vi "Measurement UI.vi"() -> ()   [LabVIEW 2025, in "CAN-LIN Raw Bus Capture UI.lvlib"]
uses:
  CAN-LIN Raw Bus Capture UI.lvlib
  Toggle.ctl
  <vilib>/gRPC/LabVIEW gRPC Library/Shared/grpcId.ctl
  Get Status.vi
  Flush Table.vi
  Create Buffer.vi
  Destroy Table Buffer.vi
  OOB gRPC Client/OOB gRPC Client.lvlib
  <vilib>/gRPC/LabVIEW gRPC Library/grpc-lvsupport-release.lvlib
panel:
  out "New root item?":bool
  in  "Tree Data":string[][](array[string])
  in  "Mapping done?":bool
  in  "Table map":map{string, i32}(c390)
  in  "XNET Sessions map":map{u32, refnum<k21>}(c390)
  in  "Tags map":map{string, bool}(c390)
  out "Valid DBC file?":bool
  out "Signals in DBC":i32
  out "Frames in DBC":i32
  in  "Frames Map":map{u32, refnum<k21>}(c390)
  in  "Signals Map":map{u32, refnum<k21>[]}(c390)
  in  "Tree and Table":enum32{"Trace window", "Signal table"}(tab)
  out "Frames":string(tree)
  out "Signals":string[][](table)
  in  "HELP":bool
  out "IsRestarting?":bool
  out "Table Buffer":i32
  out "Error (Logic)":string
  out "Status Message":string
  in  "SAVE FORMAT":u16(ring) items=["TDMS", "CSV"]
  out "Connection":bool
  in  "Clear Trace":bool
  in  "Bus Type":string="CAN"
  in  "Lin Interface":string
  in  "Can Interface":string
  in  "PauseResume":bool
  in  "Path":path
  in  "Save":bool
  in  "Filter":string
  in  "SortByID":bool
  out "Status":string
  in  "SETTINGS":enum32{"CAN", "LIN"}(tab)
  in  "IO Mode":enum32{"CAN", "CAN FD", "CAN FD + BRS"}(ring)
  in  "FD ISO Mode":enum32{"ISO", "Non ISO", "Legacy ISO"}(ring)
  in  "Baudrate":u32=125000
  in  "FD Baudrate":u32=1000000
  in  "Termination CAN":T1
  in  "INTERFACE NAME CAN":refnum<k21>
  in  "DBC path":path
  in  "Termination LIN":T1
  in  "INTERFACE NAME LIN":refnum<k21>
  out "Buffer Size":i32
  out "OOB gRPC Port":i32
  # "CONFIGURATION"
  # "CONTROL"
  # "DBC INFORMATION"
  # "STATUS"
  # "CAN Settings"
  # "LIN Settings"
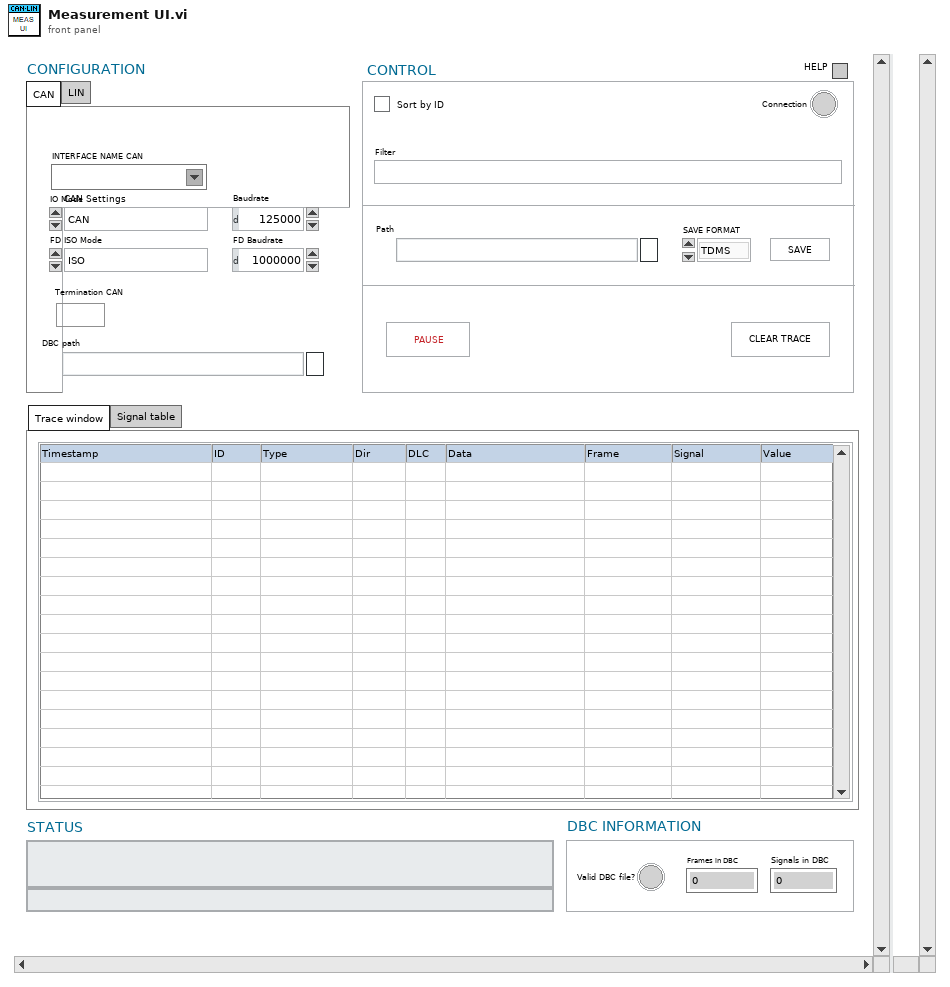
[diagram p1: front panel]
types:
  T1 = typedef "Toggle.ctl" = bool
  T2 = typedef "grpc-lvsupport-release.lvlib/grpcId.ctl" = u64
  T3 = cluster{"New root item?":refnum<vi>, "Tree Data":refnum<vi>, "Mapping done?":refnum<vi>, "Table map":refnum<vi>, "Tags map":refnum<vi>, "XNET Sessions map":refnum<vi>, "Signals":refnum<vi>, "PauseResume":refnum<vi>, "Clear Trace":refnum<vi>, "Path":refnum<vi>, "SAVE FORMAT":refnum<vi>, "Save":refnum<vi>, "Bus Type":refnum<vi>, "Filter":refnum<vi>, "SortByID":refnum<vi>, "Status Message":refnum<vi>, "Frames":refnum<vi>, "DBC path":refnum<vi>, "Signals Map":refnum<vi>, "Frames Map":refnum<vi>, "Frames in DBC":refnum<vi>, "Signals in DBC":refnum<vi>, "Valid DBC file?":refnum<vi>}
  T4 = enum32{"Page Enabled", "Page Disabled", "Page Disabled & Grayed"}
  T5 = enum8{"Enabled", "Disabled", "Disabled and Grayed Out"}
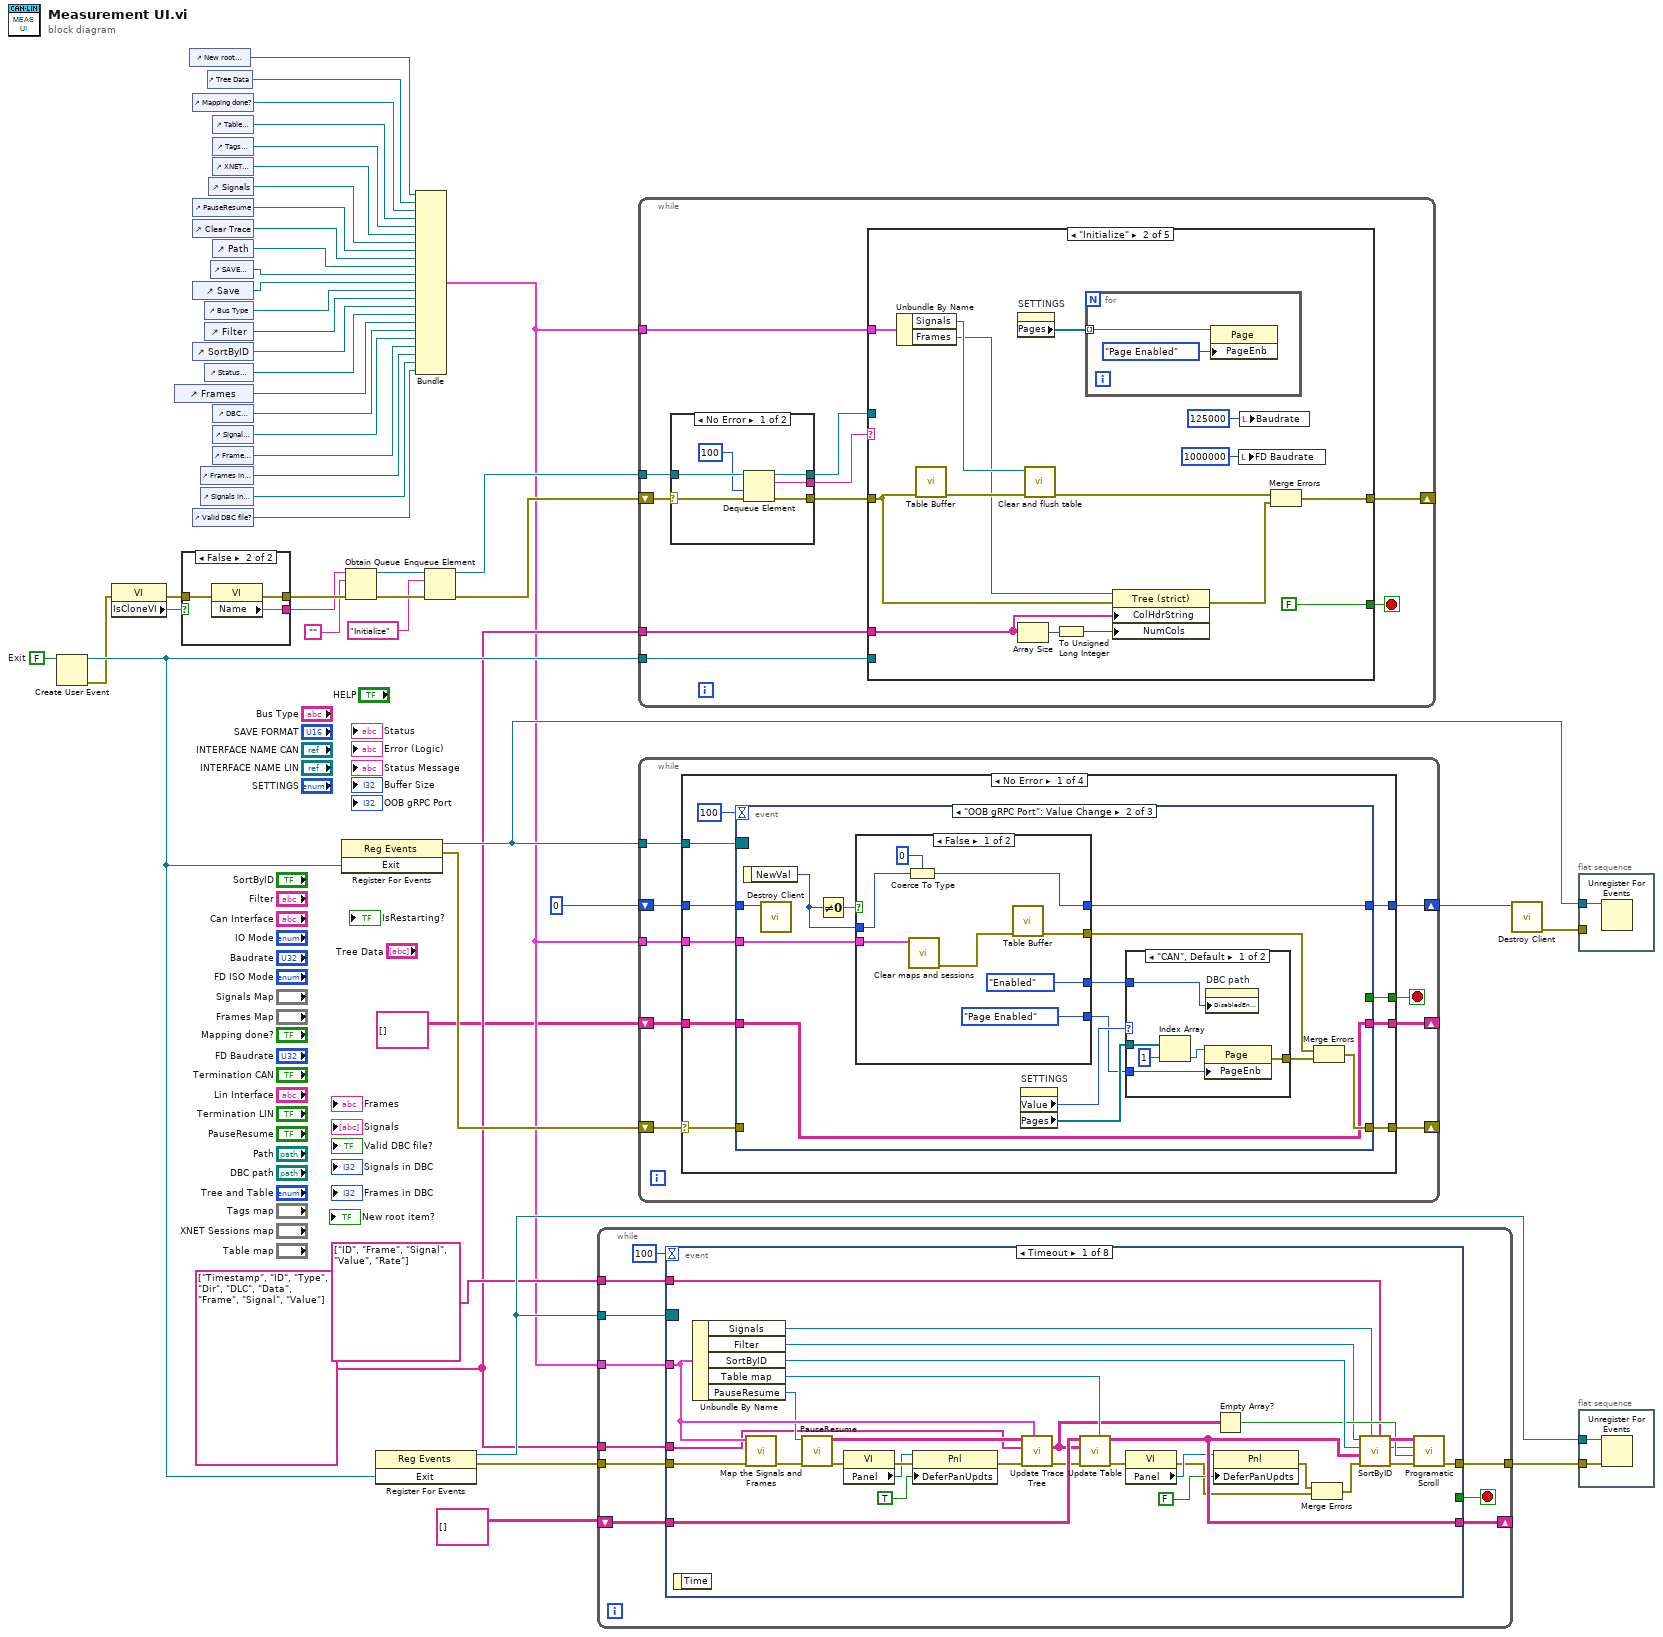
[diagram p0: block diagram]
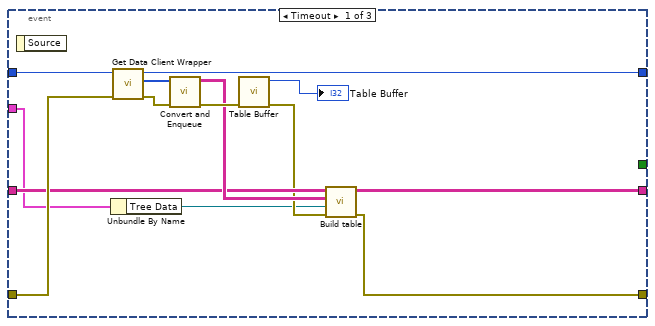
[diagram p2: hidden frame]
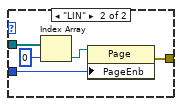
[diagram p3: hidden frame]
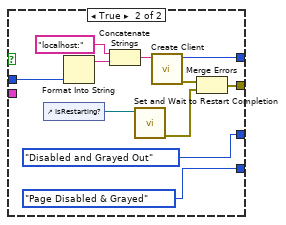
[diagram p4: hidden frame]
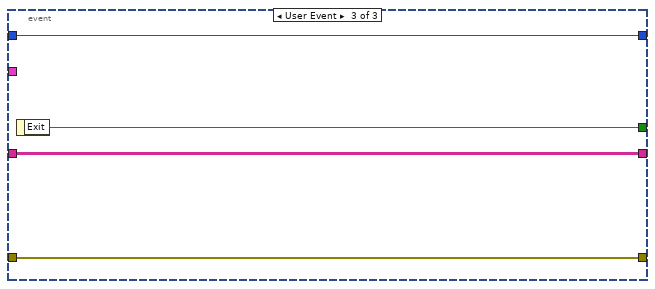
[diagram p5: hidden frame]
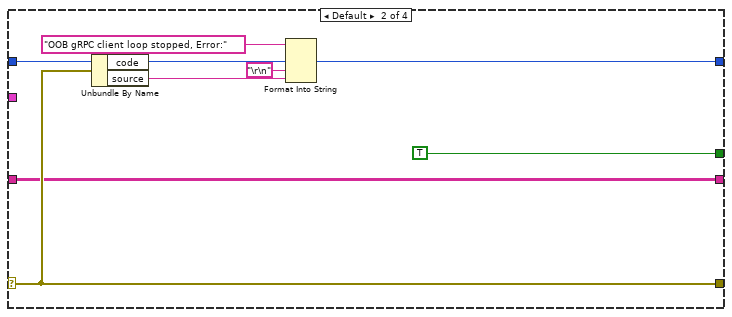
[diagram p6: hidden frame]
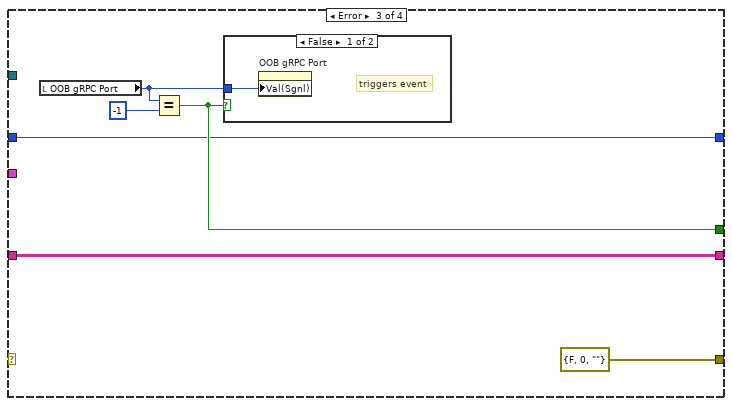
[diagram p7: hidden frame]
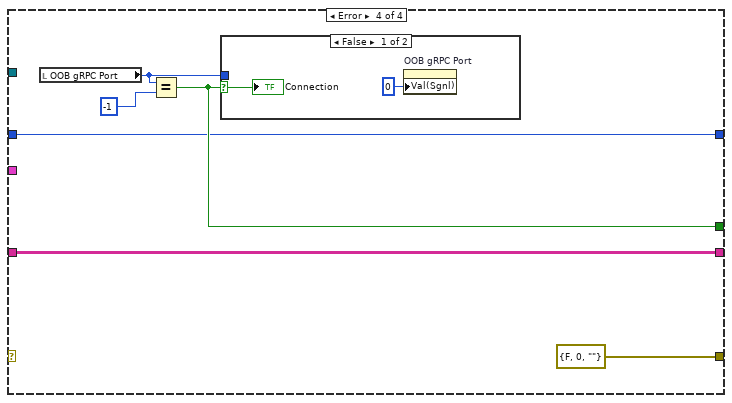
[diagram p9: hidden frame]
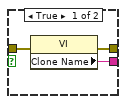
[diagram p11: hidden frame]
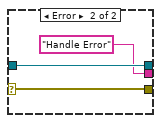
[diagram p12: hidden frame]
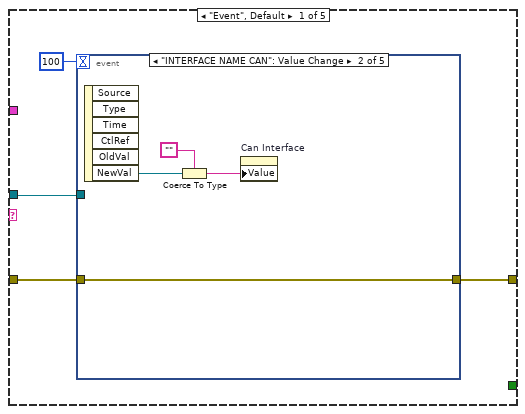
[diagram p13: hidden frame]
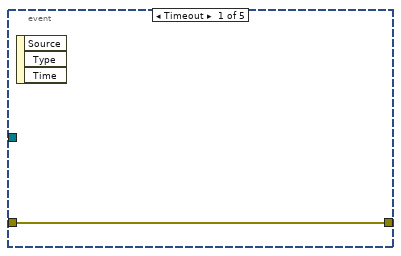
[diagram p14: hidden frame]
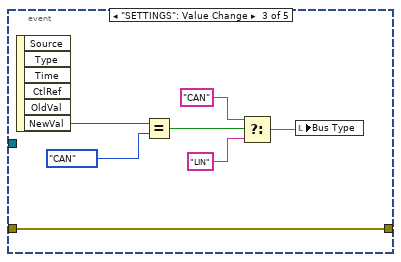
[diagram p15: hidden frame]
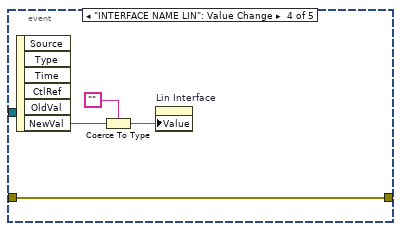
[diagram p16: hidden frame]
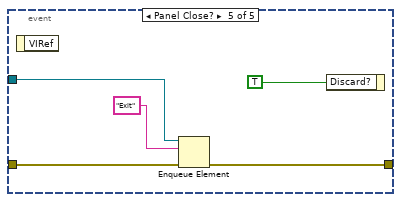
[diagram p17: hidden frame]
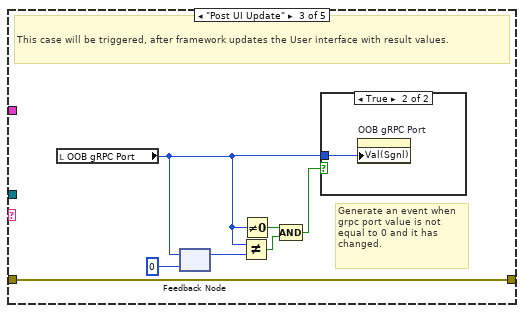
[diagram p18: hidden frame]
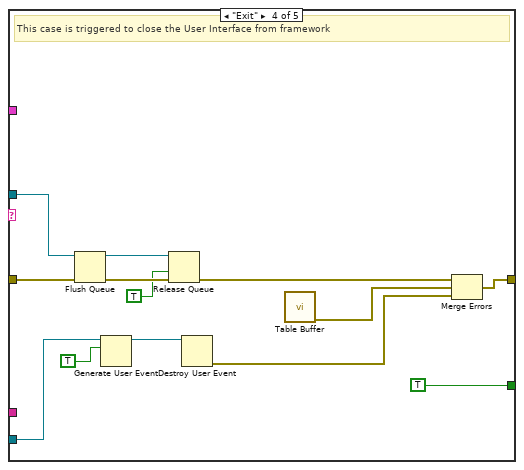
[diagram p20: hidden frame]
diagram:
  w17 = string[] ["Timestamp", "ID", "Type", "Dir", "DLC", "Data", "Frame", "Signal", "Value"] ("Headers")
  w41 = FALSE  # Exit
  n1 = Create User Event(user event datatype=w41) -> (user event=w35:refnum<user-event>, error out=w7:errorcluster)  [unwired: 1 in]
  n2 = property class="VI"(error in=w7) -> (error out=w42:errorcluster, "IsCloneVI"=w43:bool)  [unwired: 1 in, 1 out]
  n3 = control-ref of="Frames"() -> (w21:refnum<vi>)
  n4 = case shown="False" w43 {
    tunnel: [w52 w55] -> w49
    tunnel: [w51 w54] -> w48
    tunnel: w42 -> [w50 w53]
    frame True {
      n5 = property class="VI"(error in=w50) -> (error out=w52:errorcluster, "Clone Name"=w51:string)  [unwired: 1 in, 1 out]
    }
    frame False {
      n6 = property class="VI"(error in=w53) -> (error out=w55:errorcluster, "Name"=w54:string)  [unwired: 1 in, 1 out]
    }
  }
  n7 = control-ref of="New root item?"() -> (w1:refnum<vi>)
  n8 = control-ref of="Mapping done?"() -> (w5:refnum<vi>)
  n9 = control-ref of="PauseResume"() -> (w25:refnum<vi>)
  n10 = control-ref of="Clear Trace"() -> (w33:refnum<vi>)
  n11 = control-ref of="Save"() -> (w30:refnum<vi>)
  n12 = control-ref of="SortByID"() -> (w28:refnum<vi>)
  n13 = control-ref of="Valid DBC file?"() -> (w13:refnum<vi>)
  n14 = control-ref of="Frames in DBC"() -> (w15:refnum<vi>)
  n15 = control-ref of="Signals in DBC"() -> (w14:refnum<vi>)
  n16 = control-ref of="Bus Type"() -> (w29:refnum<vi>)
  n17 = control-ref of="Filter"() -> (w27:refnum<vi>)
  n18 = control-ref of="Status Message"() -> (w26:refnum<vi>)
  n19 = control-ref of="Tree Data"() -> (w2:refnum<vi>)
  n20 = control-ref of="Signals"() -> (w34:refnum<vi>)
  n21 = control-ref of="SAVE FORMAT"() -> (w31:refnum<vi>)
  n22 = control-ref of="Table map"() -> (w10:refnum<vi>)
  n23 = control-ref of="Tags map"() -> (w12:refnum<vi>)
  n24 = control-ref of="XNET Sessions map"() -> (w11:refnum<vi>)
  n25 = control-ref of="Path"() -> (w32:refnum<vi>)
  n26 = control-ref of="DBC path"() -> (w22:refnum<vi>)
  n27 = control-ref of="Signals Map"() -> (w18:refnum<vi>)
  n28 = control-ref of="Frames Map"() -> (w19:refnum<vi>)
  n29 = register-events(w35) -> (reference out=w37:refnum<event-registration>, error out=w40:errorcluster)  [unwired: 2 in]
  n30 = Obtain Queue(name (unnamed)=w48, element data type="", error in (no error)=w49) -> (queue out=w46:refnum<queue>, error out=w47:errorcluster)  [unwired: 2 in, 1 out]
  n31 = register-events(w35) -> (reference out=w24:refnum<event-registration>, error out=w8:errorcluster)  [unwired: 2 in]
  n32 = Bundle("New root item?"=w1, "Tree Data"=w2, "Mapping done?"=w5, "Table map"=w10, "Tags map"=w12, "XNET Sessions map"=w11, "Signals"=w34, "PauseResume"=w25, "Clear Trace"=w33, "Path"=w32, "SAVE FORMAT"=w31, "Save"=w30, "Bus Type"=w29, "Filter"=w27, "SortByID"=w28, "Status Message"=w26, "Frames"=w21, "DBC path"=w22, "Signals Map"=w18, "Frames Map"=w19, "Frames in DBC"=w15, "Signals in DBC"=w14, "Valid DBC file?"=w13) -> (w4:T3)  [unwired: 1 in]
  n33 = Enqueue Element(queue=w46, element="Initialize", error in (no error)=w47) -> (queue out=w16:refnum<queue>, error out=w9:errorcluster)  [unwired: 1 in, 1 out]
  n34 = while {
    tunnel: w8 -> [w65]
    tunnel: [w60] -> w6
    tunnel: w24 -> [w64]
    tunnel: w4 -> [w61]
    shift-right: [w58] -> _
    shift-left: string[][] [] ("Table Data out") -> [w59]
    tunnel: string[] ["ID", "Frame", "Signal", "Value", "Rate"] ("Signal Table Headers") -> [w57]
    tunnel: w17 -> [w56]
    stop <- w63 stop-if-true
    n35 = event shown="[0] Timeout" {
      selector: w64 -> [_ _ _ _ _ _ _ _]
      dyn-events: _ -> [_ _ _ _ _ _ _ _]
      timeout: 100 -> [_ _ _ _ _ _ _ _]
      tunnel: w65 -> [w87 w98 w117 w134 w158 w163 w173 w175]
      tunnel: [w71 w97 w116 w133 w151 w161 w172 w175] -> w60
      tunnel: [_ _ _ _ _ _ _ w176] -> w63
      tunnel: w61 -> [w85 _ w113 w135 w160 w167 _ _]
      tunnel: w59 -> [w82 w96 w108 w132 w155 w168 w171 w174]
      tunnel: [w95 w96 w109 w132 w155 w168 w171 w174] -> w58
      tunnel: w57 -> [w88 _ _ _ w154 _ _ _]
      tunnel: w56 -> [w69 _ _ w130 _ w162 _ _]
      event Timeout {
        n36 = event-data() -> ()  [unwired: 1 in, 1 out]
        n37 = Unbundle By Name(w85) -> ("Signals"=w90:refnum<vi>, "Filter"=w72:refnum<vi>, "SortByID"=w92:refnum<vi>, "Table map"=w83:refnum<vi>, "PauseResume"=w84:refnum<vi>)
        n38 = call "Map the Signals and Frames.vi"("error in"=w87, "References"=w85) -> ("error out"=w86:errorcluster)  [unwired: 9 in]
        n39 = call "PauseResume.vi"("error in"=w86, "PauseResume Ref"=w84) -> ("error out"=w80:errorcluster, "Data"=w89:string[][])  [unwired: 8 in]
        n40 = property class="VI"(error in=w80) -> (error out=w81:errorcluster, "Panel"=w77:refnum<vi>)  [unwired: 1 in, 1 out]
        n41 = property class="Pnl"(reference=w77, error in=w81, "DeferPanUpdts"=TRUE ("Defer Panel Updates")) -> (error out=w79:errorcluster)  [unwired: 1 out]
        n42 = call "Update Trace Tree.vi"("References"=w85, "error in"=w79, "Headers"=w69, "Data IN"=w89) -> ("error out"=w73:errorcluster, "Signals"=w76:string[][])  [unwired: 6 in]
        n43 = call "Update Table.vi"("Table map"=w83, "error in"=w73, "New Data in"=w76, "Table Data in"=w82) -> ("error out"=w70:errorcluster, "Table Data out"=w95:string[][])  [unwired: 6 in]
        n44 = property class="VI"(error in=w70) -> (error out=w68:errorcluster, "Panel"=w74:refnum<vi>)  [unwired: 1 in, 1 out]
        n45 = property class="Pnl"(reference=w74, "DeferPanUpdts"=FALSE ("Defer Panel Updates")) -> (error out=w67:errorcluster)  [unwired: 1 in, 1 out]
        n46 = Empty Array?(array=w76) -> (empty?=w91:bool)
        n47 = Merge Errors(w67, w68) -> (w66:errorcluster)
        n48 = call "SortByID.vi"("Headers"=w88, "Signals table"=w90, "error in"=w66, "Unsorted Data"=w95, "SortByID"=w92, "Filter"=w72) -> ("error out"=w94:errorcluster, "Table Control"=w93:string[][])  [unwired: 4 in]
        n49 = call "Programatic Scroll.vi"("error in"=w94, "Pause? (F)"=w91, "Table Ref"=w90, "Trace"=w93) -> ("error out"=w71:errorcluster)  [unwired: 7 in]
      }
      event "Clear Trace": Value Change {
        # "Run when restarting or then button is pressed down."
        n50 = event-data() -> ("NewVal"=w99:bool)  [unwired: 1 in]
        n51 = case shown="False" w99 {
          tunnel: w98 -> [w102 w103]
          tunnel: [w100 w103] -> w97
          frame False {
            n52 = property on="IsRestarting?" class="Bool (strict)"(error in=w102, "Val(Sgnl)"=FALSE ("Value (Signaling)")) -> (error out=w100:errorcluster)  [unwired: 1 in, 1 out]
          }
          frame True {
          }
        }
      }
      event "IsRestarting?": Value Change {
        n53 = event-data() -> ("NewVal"=w115:bool)  [unwired: 1 in]
        n54 = Unbundle By Name(w113) -> ("Table map"=w104:refnum<vi>, "Tags map"=w105:refnum<vi>, "Frames"=w106:refnum<vi>, "Status Message"=w110:refnum<vi>, "Signals"=w112:refnum<vi>)
        n55 = Not(x=w115) -> (.not. x?=w114:bool)
        n56 = call "Clear Table.vi"("error in"=w117, "Confirm? (F)"=w114, "Table in"=w112) -> ("error out"=w111:errorcluster, "T button?"=w107:bool)  [unwired: 7 in]
        n57 = case shown="True" w107 {
          tunnel: [w119 w128] -> w116
          tunnel: w111 -> [w119 w126]
          tunnel: w110 -> [_ w125]
          tunnel: [w118 string[][] [] ("Table Data out")] -> w109
          tunnel: w108 -> [w118 _]
          tunnel: w106 -> [_ w122]
          tunnel: w105 -> [_ w121]
          tunnel: w104 -> [_ w120]
          frame False {
          }
          frame True {
            # "Reset Table when necessary"
            n58 = invoke class="Map (strict)" method="Reinit To Default"(reference=w120) -> ()  [unwired: 2 in, 3 out]
            n59 = invoke class="Map (strict)" method="Reinit To Default"(reference=w121) -> ()  [unwired: 2 in, 3 out]
            n60 = property class="Str"(reference=w125, error in=w126, "Value"="") -> (error out=w127:errorcluster)  [unwired: 1 out]
            n61 = property on="IsRestarting?" class="Bool (strict)"(error in=w127, "Value"=FALSE ("IsRestarting?")) -> (error out=w128:errorcluster)  [unwired: 1 in, 1 out]
            n62 = invoke on="Invoke Node" class="Tree (strict)" method="Edit Tree Items.Delete"(reference=w122) -> ()  [unwired: 4 in, 5 out]
          }
        }
      }
      event "Save": Value Change {
        n63 = event-data() -> ("NewVal"=w131:bool)  [unwired: 1 in]
        n64 = case shown="False" w131 {
          tunnel: w135 -> [_ w149]
          tunnel: w134 -> [w136 w145]
          tunnel: [w136 w143] -> w133
          tunnel: w130 -> [_ w141]
          frame True {
          }
          frame False {
            n65 = Unbundle By Name(w149) -> ("DBC path"=w138:refnum<vi>, "Status Message"=w140:refnum<vi>, "Path"=w148:refnum<vi>, "SAVE FORMAT"=w147:refnum<vi>, "Bus Type"=w146:refnum<vi>, "Tree Data"=w137:refnum<vi>, "Frames"=w139:refnum<vi>)
            n66 = call "Save CAN data.vi"("Frames"=w139, "DBC path"=w138, "Tree Data"=w137, "Headers"=w141, "error in"=w145, "Bus Type"=w146, "Format"=w147, "Path"=w148) -> ("error out"=w144:errorcluster, "Status"=w142:string)  [unwired: 2 in]
            n67 = property class="Str"(reference=w140, error in=w144, "Value"=w142) -> (error out=w143:errorcluster)  [unwired: 1 out]
          }
        }
      }
      event "SortByID": Value Change {
        # "This currently only checks the sorting value change,\nmigth need to check the  Filter Value Change too."
        n68 = event-data() -> ()  [unwired: 1 in, 1 out]
        n69 = Unbundle By Name(w160) -> ("Tags map"=w150:refnum<vi>, "Frames"=w153:refnum<vi>, "Signals"=w157:refnum<vi>, "Filter"=w156:refnum<vi>, "SortByID"=w159:refnum<vi>)
        n70 = call "SortByID.vi"("Headers"=w154, "Signals table"=w157, "error in"=w158, "Unsorted Data"=w155, "SortByID"=w159, "Filter"=w156) -> ("error out"=w152:errorcluster)  [unwired: 4 in, 1 out]
        n71 = call "Order tree.vi"("Tags map"=w150, "error in"=w152, "TreeControl in"=w153) -> ("error out"=w151:errorcluster)  [unwired: 8 in]
      }
      event "Filter": Value Change {
        n72 = event-data() -> ()  [unwired: 1 in, 1 out]
        n73 = Unbundle By Name(w167) -> ("Filter"=w166:refnum<vi>, "Frames"=w165:refnum<vi>, "Tags map"=w164:refnum<vi>)
        n74 = call "Filter Tree.vi"("Headers"=w162, "error in"=w163, "Tags map"=w164, "Frames"=w165, "Filter"=w166) -> ("error out"=w161:errorcluster)  [unwired: 6 in]
      }
      event "HELP": Value Change {
        n75 = event-data() -> ("NewVal"=w170:bool)  [unwired: 1 in]
        n76 = call "Open Help PDF.vi"("error in"=w173, "NewVal"=w170, "Path after documentation"=path "CAN-LIN Raw Bus Capture.pdf") -> ("error out"=w172:errorcluster)  [unwired: 8 in]
      }
      event User Event {
        n77 = event-data() -> ("Exit"=w176:bool)  [unwired: 1 in]
      }
    }
  }
  n78 = while {
    shift-right: [w181] -> _
    shift-left: w9 -> [w186]
    tunnel: w16 -> [w184]
    tunnel: w35 -> [w179]
    tunnel: w4 -> [w178]
    tunnel: w17 -> [w177]
    stop <- w180 stop-if-true
    n79 = case shown="No Error" w186 {
      selector: w186 -> [w192 w195]
      tunnel: [w191 w195] -> w185
      tunnel: w184 -> [w190 w194]
      tunnel: [w189 w194] -> w183
      tunnel: [w188 "Handle Error"] -> w182
      frame No Error {
        n80 = Dequeue Element(queue=w190, timeout in ms (-1)=100, error in (no error)=w192) -> (queue out=w189:refnum<queue>, element=w188:string, error out=w191:errorcluster)  [unwired: 1 out]
      }
      frame Error {
      }
    }
    n81 = case shown="\"Initialize\"" w182 {
      tunnel: w185 -> [w198 w223 w238 w258 w263]
      tunnel: w183 -> [w197 _ _ w256 w262]
      tunnel: [w199 w226 w238 w247 w263] -> w181
      tunnel: [_ FALSE _ TRUE _] -> w180
      tunnel: w179 -> [_ _ _ w250 _]
      tunnel: w178 -> [_ w221 _ _ _]
      tunnel: w177 -> [_ w222 _ _ _]
      frame "Event", Default {
        n82 = event shown="[1] \"INTERFACE NAME CAN\": Value Change" {
          selector: _ -> [_ _ _ _ _]
          dyn-events: _ -> [_ _ _ _ _]
          timeout: 100 -> [_ _ _ _ _]
          tunnel: [w200 w204 w206 w215 w219] -> w199
          tunnel: w198 -> [w200 w204 w206 w215 w220]
          tunnel: w197 -> [_ _ _ _ w218]
          event Timeout {
            n83 = event-data() -> ()  [unwired: 1 in, 3 out]
          }
          event "INTERFACE NAME CAN": Value Change {
            n84 = event-data() -> ("NewVal"=w202:refnum<k21>)  [unwired: 1 in, 5 out]
            n85 = Coerce To Type(0:w202, 1:"") -> (2:w201:string)
            n86 = property on="Can Interface" class="Str"("Value"=w201) -> ()  [unwired: 2 in, 2 out]
          }
          event "SETTINGS": Value Change {
            n87 = event-data() -> ("NewVal"=w211:enum32{"CAN", "LIN"})  [unwired: 1 in, 5 out]
            n88 = Equal?(x=w211, y=enum32{"CAN", "LIN"}."CAN") -> (x = y?=w209:bool)
            n89 = Select(t="CAN", s=w209, f="LIN") -> (s? t:f=w205:string)
            n90 = local write "Bus Type"(w205) -> ()
          }
          event "INTERFACE NAME LIN": Value Change {
            n91 = event-data() -> ("NewVal"=w212:refnum<k21>)  [unwired: 1 in, 5 out]
            n92 = Coerce To Type(0:w212, 1:"") -> (2:w213:string)
            n93 = property on="Lin Interface" class="Str"("Value"=w213) -> ()  [unwired: 2 in, 2 out]
          }
          event Panel Close? {
            n94 = event-data() -> ()  [unwired: 1 in, 1 out]
            n95 = Enqueue Element(queue=w218, element="Exit", error in (no error)=w220) -> (error out=w219:errorcluster)  [unwired: 1 in, 2 out]
            n96 = event-data("Discard?"=TRUE) -> ()  [unwired: 1 in, 1 out]
          }
        }
      }
      frame "Initialize" {
        n97 = Unbundle By Name(w221) -> ("Signals"=w232:refnum<vi>, "Frames"=w227:refnum<vi>)
        n98 = call-poly "Table Buffer.vi"("error in (no error)"=w223) -> ("error out"=w230:errorcluster)  [unwired: 10 in]
        n99 = property on="SETTINGS" class="TabCtl (strict)"() -> ("Pages"=w231:refnum<vi>[])  [unwired: 2 in, 2 out]
        n100 = Array Size(array=w222) -> (size(s)=w228:i32)
        n101 = call "Clear and flush table.vi"("error in"=w230, "Trace"=w232) -> ("error out"=w225:errorcluster)  [unwired: 9 in]
        n102 = To Unsigned Long Integer(number=w228) -> (unsigned 32bit integer=w229:u32)
        n103 = for {
          tunnel: w231 -> [w237] mode=indexing
          n104 = property class="Page"(reference=w237, "PageEnb"=T4."Page Enabled" ("Page Enabled State")) -> ()  [unwired: 1 in, 2 out]
        }
        n105 = property on="Property Node" class="Tree (strict)"(reference=w227, error in=w223, "ColHdrString"=w222, "NumCols"=w229) -> (error out=w224:errorcluster)  [unwired: 1 out]
        n106 = local write "FD Baudrate"(u32 1000000 ("FD Baudrate")) -> ()
        n107 = local write "Baudrate"(u32 125000 ("Baudrate")) -> ()
        n108 = Merge Errors(w225, w224) -> (w226:errorcluster)
      }
      frame "Post UI Update" {
        # "Generate an event when grpc port value is not equal to 0 and it has changed."
        # "This case will be triggered, after framework updates the User interface with result values."
        n109 = local read "OOB gRPC Port"() -> (w241:i32)
        n110 = feedback #1(0 ("OOB gRPC Port")) -> (w240:i32)
        n111 = feedback-in #1(w241) -> ()
        n112 = Not Equal?(x=w241, y=w240) -> (x != y?=w242:bool)
        n113 = Not Equal To 0?(x=w241) -> (x != 0?=w243:bool)
        n114 = Compound Arithmetic op=AND(w243, w242) -> (w239:bool)
        n115 = case shown="True" w239 {
          tunnel: w241 -> [_ w245]
          frame False {
          }
          frame True {
            n116 = property on="OOB gRPC Port" class="DigNum (strict)"("Val(Sgnl)"=w245) -> ()  [unwired: 2 in, 2 out]
          }
        }
      }
      frame "Exit" {
        # "This case is triggered to close the User Interface from framework"
        n117 = Flush Queue(queue=w256, error in (no error)=w258) -> (queue out=w255:refnum<queue>, error out=w254:errorcluster)  [unwired: 1 out]
        n118 = Generate User Event(user event=w250, event data cluster=TRUE ("event data")) -> (user event out=w252:refnum<user-event>)  [unwired: 2 in, 1 out]
        n119 = Release Queue(queue=w255, force destroy? (F)=TRUE, error in (no error)=w254) -> (error out=w246:errorcluster)  [unwired: 2 out]
        n120 = Destroy User Event(user event=w252) -> (error out=w249:errorcluster)  [unwired: 1 in]
        n121 = call-poly "Table Buffer.vi"() -> ("error out"=w248:errorcluster)  [unwired: 11 in]
        n122 = Merge Errors(w246, w248, w249) -> (w247:errorcluster)
      }
      frame "Handle Error" {
        w261 = "UI main loop stopped, Error: %d - %s" ("format string")
        n123 = Unbundle By Name(w263) -> ("code"=w264:i32, "source"=w259:string)
        n124 = case shown="Default" w263 {
          selector: w263 -> [w265 w270]
          tunnel: [w265 w269] -> _
          tunnel: w262 -> [_ w266]
          frame No Error {
          }
          frame Default {
            n125 = call <vilib>:"Clear Errors.vi"("error in (no error)"=w270) -> ("error out"=w268:errorcluster)  [unwired: 5 in, 1 out]
            n126 = Enqueue Element At Opposite End(queue=w266, element="Exit", error in (no error)=w268) -> (error out=w269:errorcluster)  [unwired: 1 in, 2 out]
          }
        }
        n127 = Format Into String(format string=w261, initial string=w261, w264, w259) -> (resulting string=w260:string)  [unwired: 1 in, 1 out]
        n128 = local write "Status Message"(w260) -> ()
      }
    }
  }
  n129 = while {
    tunnel: w37 -> [w276]
    shift-right: [w277] -> _
    shift-left: w40 -> [w279]
    shift-right: [w274] -> w38
    shift-left: T2 0 ("gRPC ID out") -> [w275]
    tunnel: w4 -> [w273]
    shift-right: [w271] -> _
    shift-left: string[][] [] ("Table Data in") -> [w272]
    stop <- w278 stop-if-true
    n130 = case shown="No Error" w279 {
      selector: w279 -> [w287 w352 _ _]
      tunnel: [w284 TRUE w362 w369] -> w278
      tunnel: [w288 w352 errorcluster {"status"=FALSE, "code"=0, "source"=""} ("error IO") errorcluster {"status"=FALSE, "code"=0, "source"=""} ("error IO")] -> w277
      tunnel: w276 -> [w289 _ _ _]
      tunnel: w275 -> [w286 w357 w361 w368]
      tunnel: [w285 w357 w361 w368] -> w274
      tunnel: w273 -> [w282 _ _ _]
      tunnel: w272 -> [w281 w351 w359 w366]
      tunnel: [w280 w351 w359 w366] -> w271
      frame No Error {
        n131 = event shown="[1] \"OOB gRPC Port\": Value Change" {
          selector: w289 -> [_ _ _]
          dyn-events: _ -> [_ _ _]
          timeout: 100 -> [_ _ _]
          tunnel: [w293 w307 w348] -> w288
          tunnel: w287 -> [w297 _ w348]
          tunnel: w286 -> [w298 w316 w349]
          tunnel: [w303 w315 w349] -> w285
          tunnel: [_ _ w350] -> w284
          tunnel: w282 -> [w291 w305 _]
          tunnel: w281 -> [w295 w304 w347]
          tunnel: [w292 w304 w347] -> w280
          event Timeout {
            n132 = event-data() -> ()  [unwired: 1 in, 1 out]
            n133 = Unbundle By Name(w291) -> ("Tree Data"=w290:refnum<vi>)
            n134 = call "Get Data Client Wrapper.vi"("error in"=w297, "gRPC ID in"=w298) -> ("error out"=w302:errorcluster, "Payload"=w301:u8[], "gRPC ID out"=w303:T2)  [unwired: 7 in]
            n135 = call "Convert and Enqueue.vi"("error in"=w302, "Data"=w301) -> ("error out"=w300:errorcluster, "Table Data"=w296:string[][])  [unwired: 8 in]
            n136 = call-poly "Table Buffer.vi"("error in"=w300) -> ("error out"=w294:errorcluster, "Messages"=→"Table Buffer":i32)  [unwired: 9 in]
            n137 = call "Build table.vi"("error in"=w294, "Tree Data"=w290, "New Data in"=w296, "Tree Data in"=w295) -> ("error out"=w293:errorcluster, "Tree Data out"=w292:string[][])  [unwired: 6 in]
          }
          event "OOB gRPC Port": Value Change {
            n138 = event-data() -> ("NewVal"=w313:i32)  [unwired: 1 in]
            n139 = call "Destroy Client.vi"("gRPC ID"=w316) -> ()  [unwired: 10 in, 1 out]
            n140 = Not Equal To 0?(x=w313) -> (x != 0?=w314:bool)
            n141 = case shown="False" w314 {
              tunnel: [w331 w339] -> w308
              tunnel: w313 -> [w334 w343]
              tunnel: [w332 w342] -> w315
              tunnel: [T4."Page Enabled" ("Page Enabled State") T4."Page Disabled & Grayed" ("Page Enabled State")] -> w310
              tunnel: [T5."Enabled" ("DisabledEnum") T5."Disabled and Grayed Out" ("DisabledEnum")] -> w306
              tunnel: w305 -> [w329 _]
              frame False {
                n142 = Coerce To Type(0:w334, 1:T2 0 ("gRPC ID Out")) -> (2:w332:T2)
                n143 = call "Clear maps and sessions.vi"("References"=w329) -> ("error out"=w328:errorcluster)  [unwired: 10 in]
                n144 = call-poly "Table Buffer.vi"("error in"=w328) -> ("error out"=w331:errorcluster)  [unwired: 10 in]
              }
              frame True {
                n145 = control-ref of="IsRestarting?"() -> (w337:refnum<vi>)
                n146 = Format Into String(w343) -> (resulting string=w346:string)  [unwired: 3 in, 1 out]
                n147 = Concatenate Strings("localhost:" ("string"), w346) -> (w344:string)
                n148 = call "Set and Wait to Restart Completion.vi"("Bool Ref"=w337) -> ("error out"=w338:errorcluster)  [unwired: 10 in]
                n149 = call "Create Client.vi"("address"=w344) -> ("error out"=w340:errorcluster, "gRPC ID Out"=w342:T2)  [unwired: 9 in]
                n150 = Merge Errors(w340, w338) -> (w339:errorcluster)
              }
            }
            n151 = property on="SETTINGS" class="TabCtl (strict)"() -> ("Value"=w312:enum32{"CAN", "LIN"}, "Pages"=w311:refnum<vi>[])  [unwired: 2 in, 2 out]
            n152 = case shown="\"CAN\", Default" w312 {
              tunnel: w311 -> [w322 w327]
              tunnel: w310 -> [w319 w325]
              tunnel: [w318 w323] -> w309
              tunnel: w306 -> [w317 _]
              frame "CAN", Default {
                n153 = Index Array(array=w322, index=1) -> (element=w320:refnum<vi>)
                n154 = property class="Page"(reference=w320, "PageEnb"=w319) -> (error out=w318:errorcluster)  [unwired: 1 in, 1 out]
                n155 = property on="DBC path" class="Path"("DisabledEnum"=w317) -> ()  [unwired: 2 in, 2 out]
              }
              frame "LIN" {
                n156 = Index Array(array=w327, index=0) -> (element=w326:refnum<vi>)
                n157 = property class="Page"(reference=w326, "PageEnb"=w325) -> (error out=w323:errorcluster)  [unwired: 1 in, 1 out]
              }
            }
            n158 = Merge Errors(w308, w309) -> (w307:errorcluster)
          }
          event User Event {
            n159 = event-data() -> ("Exit"=w350:bool)  [unwired: 1 in]
          }
        }
      }
      frame Default {
        n160 = Unbundle By Name(w352) -> ("code"=w356:i32, "source"=w355:string)
        n161 = Format Into String(initial string="OOB gRPC client loop stopped, Error:" ("format string"), w356, "\r\n", w355) -> ()  [unwired: 2 in, 2 out]
      }
      frame Error {
        n162 = local read "OOB gRPC Port"() -> (w364:i32)
        n163 = Equal?(x=w364, y=-1 ("x")) -> (x = y?=w362:bool)
        n164 = case shown="False" w362 {
          tunnel: w364 -> [w365 _]
          frame False {
            # "triggers event"
            n165 = property on="OOB gRPC Port" class="DigNum (strict)"("Val(Sgnl)"=w365) -> ()  [unwired: 2 in, 2 out]
          }
          frame True {
          }
        }
      }
      frame Error {
        n166 = local read "OOB gRPC Port"() -> (w371:i32)
        n167 = Equal?(x=w371, y=-1 ("x")) -> (x = y?=w369:bool)
        n168 = case shown="False" w369 {
          selector: w369 -> [w372 _]
          tunnel: w371 -> [_ _]
          frame False {
            n169 = property on="OOB gRPC Port" class="DigNum (strict)"("Val(Sgnl)"=0 ("Value (Signaling)")) -> ()  [unwired: 2 in, 2 out]
            "Connection" <- w372
          }
          frame True {
          }
        }
      }
    }
  }
  n170 = call "Destroy Client.vi"("gRPC ID"=w38) -> ("error out"=w39:errorcluster)  [unwired: 10 in]
  n171 = flat-sequence {
    tunnel: w37 -> [w374]
    tunnel: w39 -> [_]
    frame #0 {
      n172 = Unregister For Events(event registration refnum=w374) -> ()  [unwired: 1 in, 1 out]
    }
  }
  n173 = flat-sequence {
    tunnel: w24 -> [w376]
    tunnel: w6 -> [w375]
    frame #0 {
      n174 = Unregister For Events(event registration refnum=w376, error in=w375) -> ()  [unwired: 1 out]
    }
  }
